vi "Init.vi"(8 "Error Input":errorcluster, 10 "ApiKey":string, 11 "BaseUrl":string) -> (0 "Error Output":errorcluster, 3 "LiteAgentSDK Output":refnum<k24>)   [LabVIEW 2017, in "LiteAgentSDK.lvlib"]
uses:
  LiteAgentSDK.lvlib
  C:/Users/Jan/Projects/LiteAgentSDK-LabVIEW/Source/Bin/LiteAgentSDK.LabVIEW.dll
  Bin/LiteAgentSDK.LabVIEW.dll
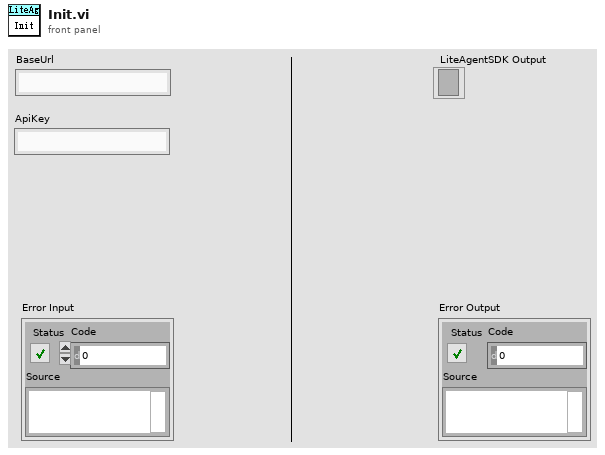
[diagram p1: front panel]
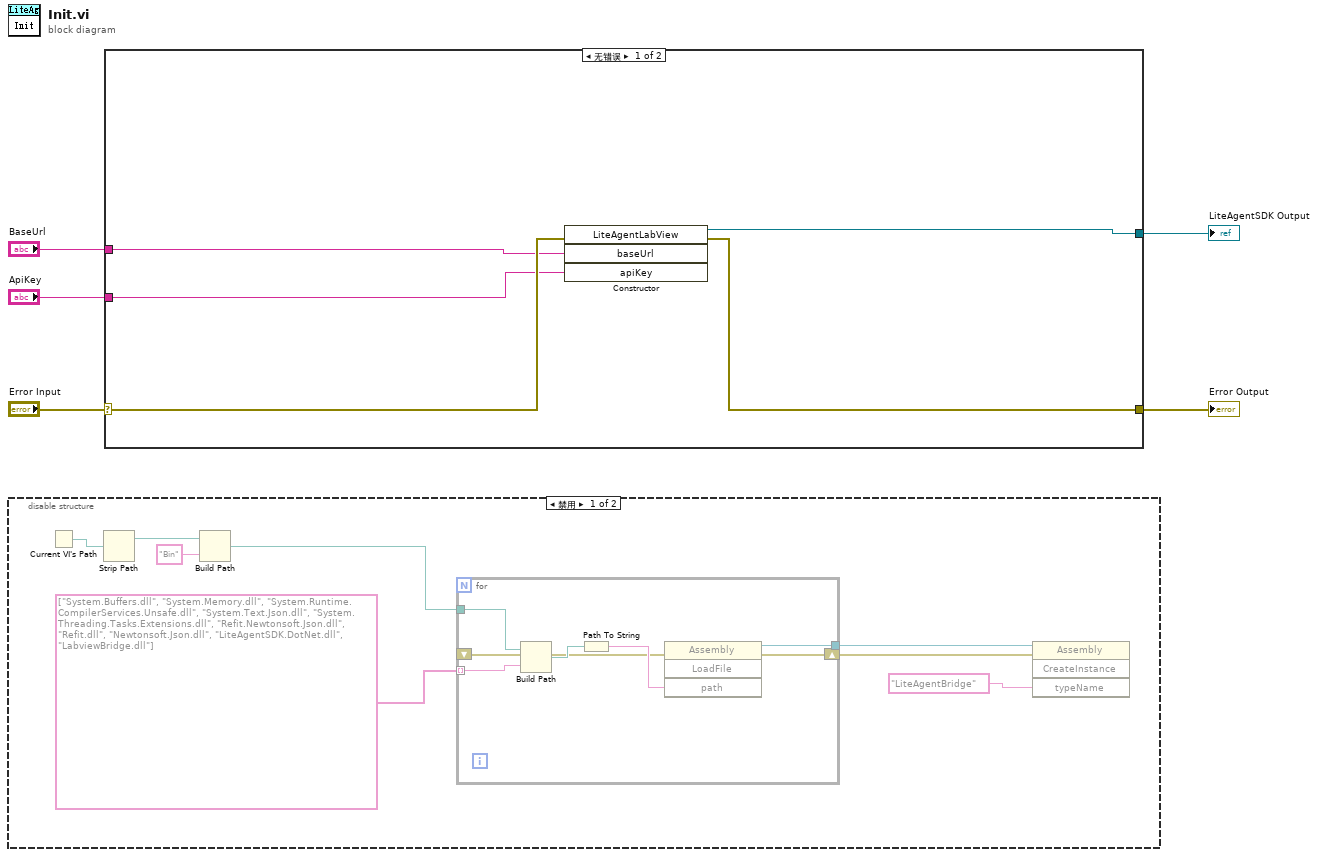
[diagram p0: block diagram]
diagram:
  n1 = disable-structure shown="禁用" {
    frame Disabled {
      n2 = Current VI's Path() -> (path=w13:path)
      n3 = Strip Path(path=w13) -> (stripped path=w12:path)  [unwired: 1 out]
      n4 = Build Path(base path=w12, name or relative path="Bin" ("名称或相对路径")) -> (appended path=w10:path)
      n5 = for {
        tunnel: string[] ["System.Buffers.dll", "System.Memory.dll", "System.Runtime.CompilerServices.Unsafe.dll", "System.Text.Json.dll", "System.Threading.Tasks.Extensions.dll", "Refit.Newtonsoft.Json.dll", "Refit.dll", "Newtonsoft.Json.dll", "LiteAgentSDK.DotNet.dll", "LabviewBridge.dll"] -> [w19] mode=indexing
        tunnel: w10 -> [w20]
        shift-right: [w15] -> w7
        shift-left: _ -> [w16]
        tunnel: [w14] -> w8
        n6 = Build Path(base path=w20, name or relative path=w19) -> (appended path=w17:path)
        n7 = Path To String(path=w17) -> (string=w18:string)
        n8 = invoke on="调用节点" class="Assembly" method="LoadFile"(error in=w16, "path"=w18) -> (reference out=w14:refnum<k24>, error out=w15:errorcluster)  [unwired: 2 in, 2 out]
      }
      n9 = invoke on="调用节点" class="Assembly" method="CreateInstance"(reference=w8, error in=w7, "typeName"="LiteAgentBridge") -> ()  [unwired: 1 in, 4 out]
    }
    frame Enabled {
    }
  }
  n10 = case shown="无错误" "Error Input" {
    selector: "Error Input" -> [w25 w26]
    tunnel: [w23 w26] -> w4
    tunnel: [w24 _] -> w3
    tunnel: "BaseUrl" -> [w22 _]
    tunnel: "ApiKey" -> [w21 _]
    frame No Error {
      n11 = constructor class="LiteAgentLabView" ("构造器节点")(error in=w25, "baseUrl"=w22, "apiKey"=w21) -> (reference out=w24:refnum<k24>, error out=w23:errorcluster)  [unwired: 2 in, 3 out]
    }
    frame Error {
    }
  }
  "Error Output" <- w4
  "LiteAgentSDK Output" <- w3
